vi "8（串口数据发送）.vi"() -> ()   [LabVIEW 2017]
uses:
  <vilib>/Instr/_visa.llb/VISA Configure Serial Port (Instr).vi
  <vilib>/Analysis/NI_AALBase.lvlib
panel:
  out "波形图表":dbl[](graph)
  in  "停止":bool
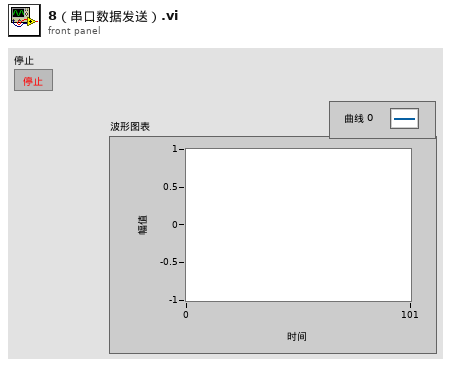
[diagram p1: front panel]
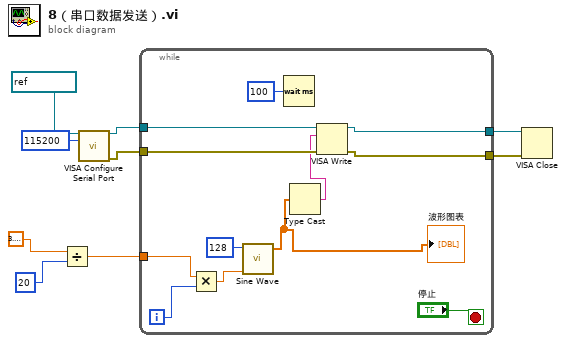
[diagram p0: block diagram]
diagram:
  n1 = Divide(x=3.141592653589793, y=20) -> (x/y=w1:dbl)
  n2 = call-poly "VISA Configure Serial Port"("VISA resource name"=refnum<visa-resource-name> "COM1", "baud rate (9600)"=u32 115200) -> ("VISA resource name out"=w7:refnum<visa-resource-name>, "error out"=w6:errorcluster)  [unwired: 12 in]
  n3 = while {
    tunnel: w7 -> [w21]
    tunnel: w6 -> [w20]
    tunnel: [w19] -> w5
    tunnel: [w18] -> w4
    tunnel: w1 -> [w15]
    i -> [w14]
    stop <- "停止" stop-if-true
    n4 = Multiply(x=w15, y=w14) -> (x*y=w13:dbl)
    n5 = call <vilib>:"Sine Wave.vi"("samples"=128, "phase in"=w13) -> ("sine wave"=w10:dbl[])  [unwired: 3 in, 2 out]
    "波形图表" <- w10
    n6 = Wait (ms)(milliseconds to wait=u32 100 ("等待时间（毫秒）")) -> ()  [unwired: 1 out]
    n7 = Type Cast(x=w10) -> (*(type *) &x=w11:string)  [unwired: 1 in]
    n8 = VISA Write(VISA resource name=w21, write buffer=w11, error in (no error)=w20) -> (VISA resource name out=w19:refnum<visa-resource-name>, error out=w18:errorcluster)  [unwired: 1 out]
  }
  n9 = VISA Close(VISA resource name=w5, error in (no error)=w4) -> ()  [unwired: 1 out]
